vi "Display name.vi"(1 "State In":T1) -> (0 "Name":string)   [LabVIEW 2018, in "Array Dimension Array.xnode"]
uses:
  Array Dimension Array.xnode
  State.ctl
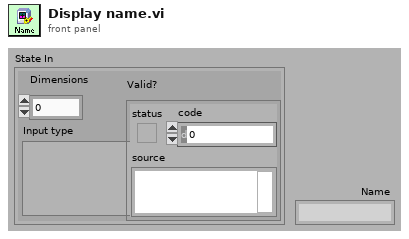
[diagram p1: front panel]
types:
  T1 = typedef "Array Dimension Array.xnode/State.ctl" = cluster{"Input type":variant, "Valid?":errorcluster, "Dimensions":i32}
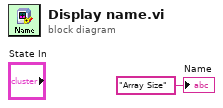
[diagram p0: block diagram]
diagram:
  "Name" <- "Array Size" ("Name")
